vi "Vision Processing.vi"(8 "error in (no error)":errorcluster, 11 "Image Size":T1=enum."320x240") -> ()   [LabVIEW 2017]
uses:
  Vision Support Code/Camera Types.ctl
  <vilib>/Rock Robotics/WPI/Camera/WPI_CameraImageSize.ctl
  <vilib>/Rock Robotics/WPI/Camera/WPI_CameraWhite Balance Values.ctl
  <vilib>/Rock Robotics/WPI/Camera/WPI_CameraExposure Values.ctl
  <vilib>/Rock Robotics/WPI/Camera/WPI_CameraFrameRate.ctl
  Robot Global Data.vi
  <vilib>/Rock Robotics/Network Tables/NT Write Number.vi
  <vilib>/vision/NI_Vision_Development_Module.lvlib
panel:
  in  "max ratio":dbl=8.0 format="%#_13g"
  in  "min ratio":dbl=3.0 format="%#_13g"
  out "error out":errorcluster
  in  "format string":string="USB 0"
  in  "Min Component %":dbl=15.0
  out "loop ms":u32
  in  "Display Original":bool
  in  "Display Mask":bool
  out "Instructions:":string="Connect a USB or IP camera to your roboRIO. If using a ring light and retroreflective tape, use Camera Settings outside the loop create a dark image with bright and colorful stripes. If used wihtout a ring light, brighten the images so that stripes are visible.\n\nLED Color can encoded as HSL or related color modes. Calibrate to the same color as the strips being reflected to the camera. Unlike the desktop example, this LED color must be set by hand. You can also put the calibration on the dashboard and send the LED Color to the RT code using Network Tables.\n\nThe Display buttons affects whether images are displayed on the panel. It takes quite a bit of CPU  to compress and transmit the images for display.\n\nAdjust Score Cutoff to make the code more or less picky. If the color is not very unique, you may need to increase the number of particles considered. The diagram uses a Size Limit to ignore colored things that are too small. You may need to adjust it if you are targetting from far away.\n\nResults give you the distance to the target, the center and box in a normalized (-1 to 1) and pixel coordinates.\n\nBe sure to read about setting camera exposure and brightness to help simplify your image and acquire color saturated images.\n\nThere are lots of comments on the diagram to explain the code."
  in  "Color Mode":u16(ring)=2 items=["RGB", "HSL", "HSV", "HSI"]
  in  "Particles":dbl=5.0
  in  "Score Cutoff %":dbl=75.0
  in  "Camera Type":T2=enum."MS HD3000 square"
  out "Result":T3 {"Score" format="%#_3g"; "Pixels"."Rectangle"."Numeric 5" format="%#_3g"; "Pixels"."Rectangle"."Numeric 3" format="%#_3g"; "Pixels"."Rectangle"."Numeric 2" format="%#_3g"; "Pixels"."Rectangle"."Numeric" format="%#_3g"; "Normalized"."Rectangle"."Numeric 5" format="%#_2g"; "Normalized"."Rectangle"."Numeric 3" format="%#_2g"; "Normalized"."Rectangle"."Numeric 2" format="%#_2g"; "Normalized"."Rectangle"."Numeric" format="%#_2g"; "Normalized"."Center"."?" format="%#_3g"; "Normalized"."Center"."?" format="%#_3g"; "Distance (ft)" format="%#_3g"}
  out "Qualified Particles":i32
  in  "LED Color":T4={"Hue"={107.81818389892578, 139.81818389892578}, "Sat"={176.07142857142858, 255.0}, "Val"={40.53571428571429, 255.0}} {"Hue" scale=0.0..255.0 scale format="%#_3g"}
  out "Mask":T5(plugin-control)
  out "Original Image":T5(plugin-control)
  # "Good target, distance ft"
  # "Bad target"
  # "Score in %"
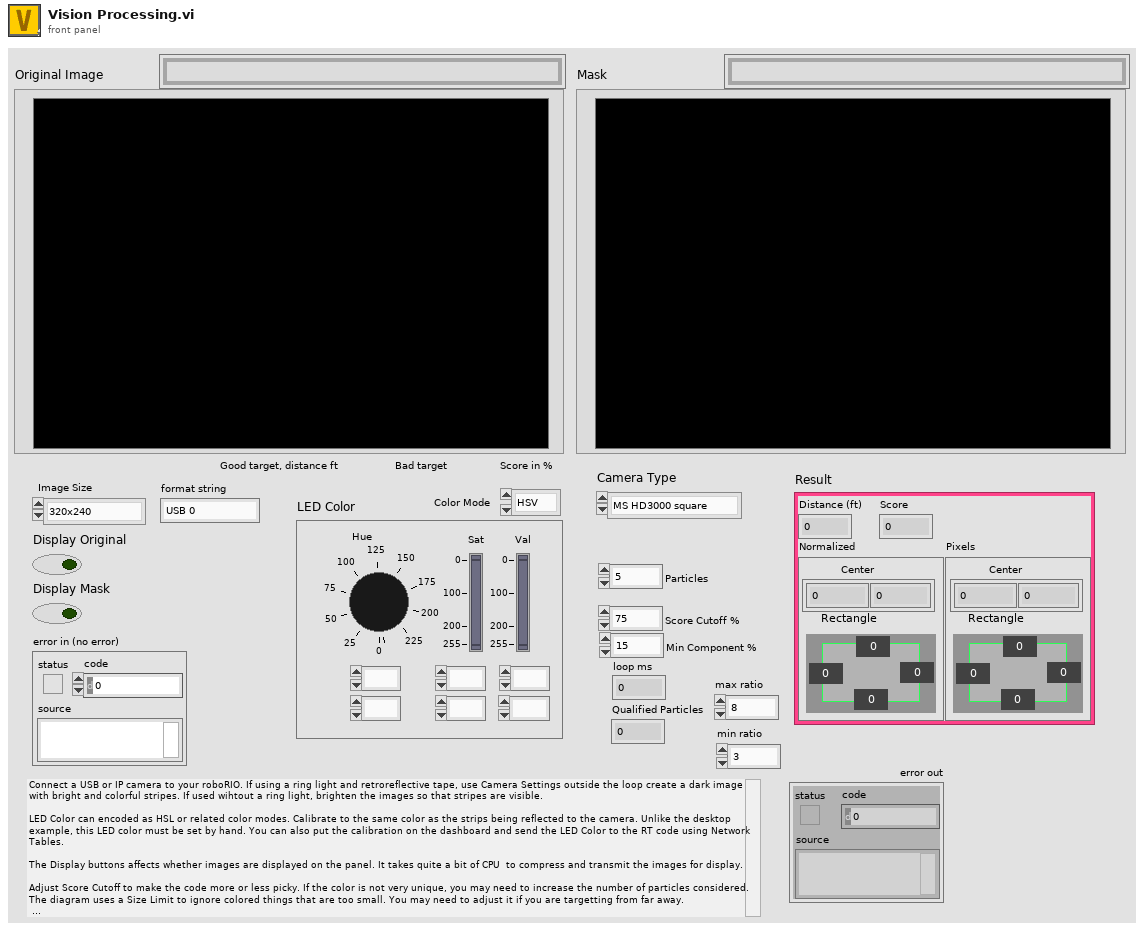
[diagram p1: front panel]
types:
  T1 = typedef "WPI_CameraImageSize.ctl" = enum16{"640x480", "320x240", "160x120", "Custom"}
  T2 = typedef "Camera Types.ctl" = enum16{"206", "1011", "1013", "MS HD3000 square", "MS HD3000 640x480"}
  T3 = cluster{"Distance (ft)":dbl, "Score":dbl, "Normalized":cluster{"Center":cluster{dbl, dbl}, "Rectangle":cluster{"Numeric":dbl, "Numeric 2":dbl, "Numeric 3":dbl, "Numeric 5":dbl}}, "Pixels":cluster{"Center":cluster{dbl, dbl}, "Rectangle":cluster{"Numeric":dbl, "Numeric 2":dbl, "Numeric 3":dbl, "Numeric 5":dbl}}}
  T4 = cluster{"Hue":cluster{dbl, dbl}, "Sat":cluster{dbl, dbl}, "Val":cluster{dbl, dbl}}
  T5 = typedef "IMAQ Image.ctl" = refnum<image>
  T6 = typedef "WPI_CameraFrameRate.ctl" = u32
  T7 = typedef "WPI_CameraExposure Values.ctl" = enum16{"Auto", "Flicker-free 50 Hz", "Flicker-free 60 Hz", "Hold current", "Custom"}
  T8 = typedef "WPI_CameraWhite Balance Values.ctl" = enum16{"Auto", "Fixed indoor", "Fixed outdoor 1", "Fixed outdoor 2", "Fixed fluorescent 1", "Fixed fluorescent 2", "Hold current", "Custom"}
  T9 = typedef "Particle Parameters" = i32
  T10 = typedef "Image Type" = u32
  T11 = typedef "WPI_CameraDevRef.ctl" = cluster{"Camera Address":string, "CameraStatus":errorcluster}
  T12 = cluster{"Score":dbl, "Rect":cluster{"Left":dbl, "Top":dbl, "Right":dbl, "Bottom":dbl}, "Full Scores":cluster{"Aspect Ratio":dbl, "Top Position":dbl, "Bottom Position":dbl, "Left Gap":dbl, "Width":dbl, "Height Ratio":dbl}}[]
  T13 = cluster{"Score":dbl, "Rect":cluster{"Left":dbl, "Top":dbl, "Right":dbl, "Bottom":dbl}, "Full Scores":cluster{"Aspect Ratio":dbl, "Top Position":dbl, "Bottom Position":dbl, "Left Gap":dbl, "Width":dbl, "Height Ratio":dbl}}
  T14 = cluster{"Left":dbl, "Top":dbl, "Right":dbl, "Bottom":dbl}
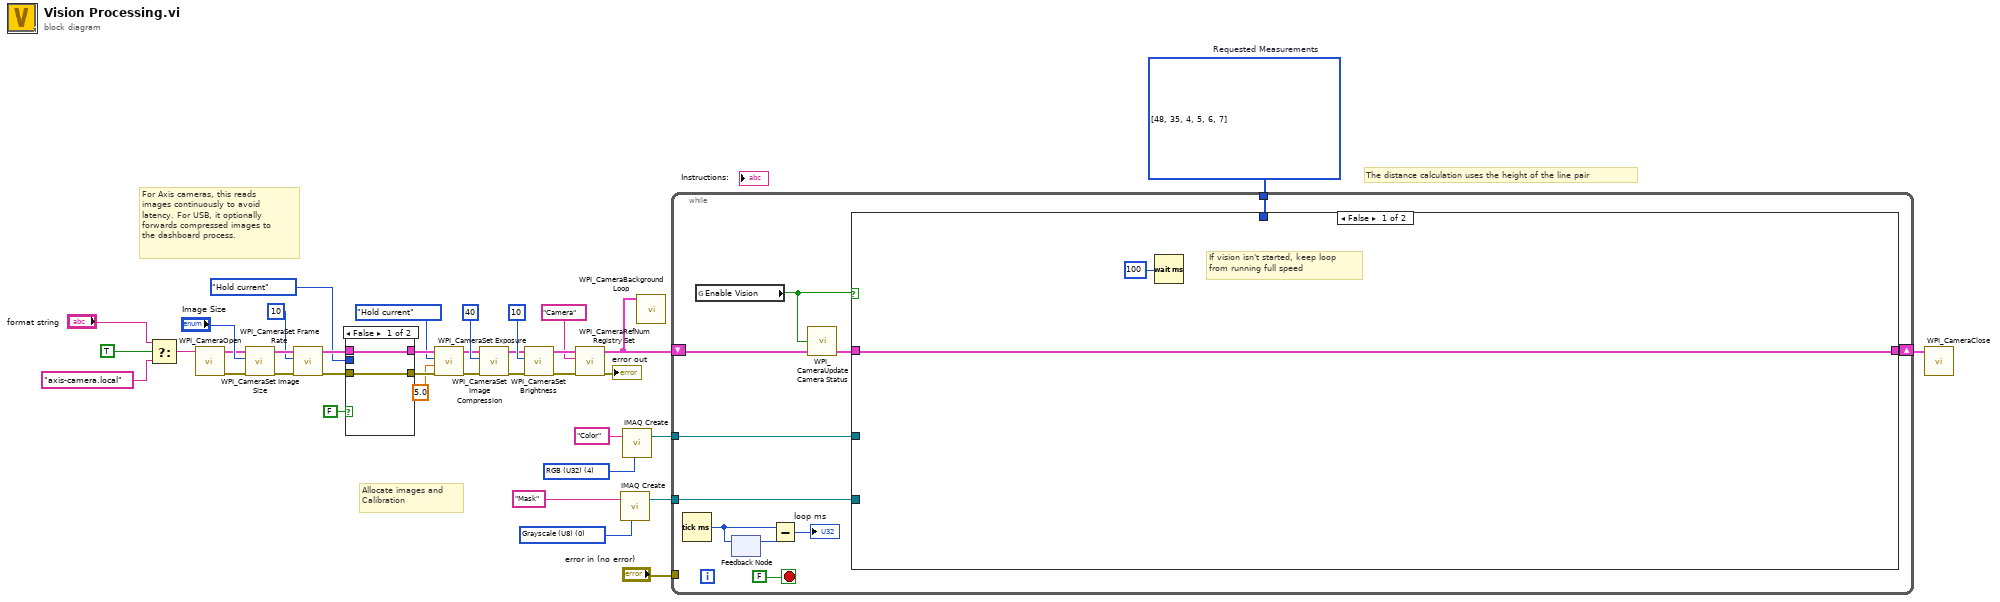
[diagram p0: block diagram]
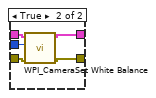
[diagram p2: hidden frame]
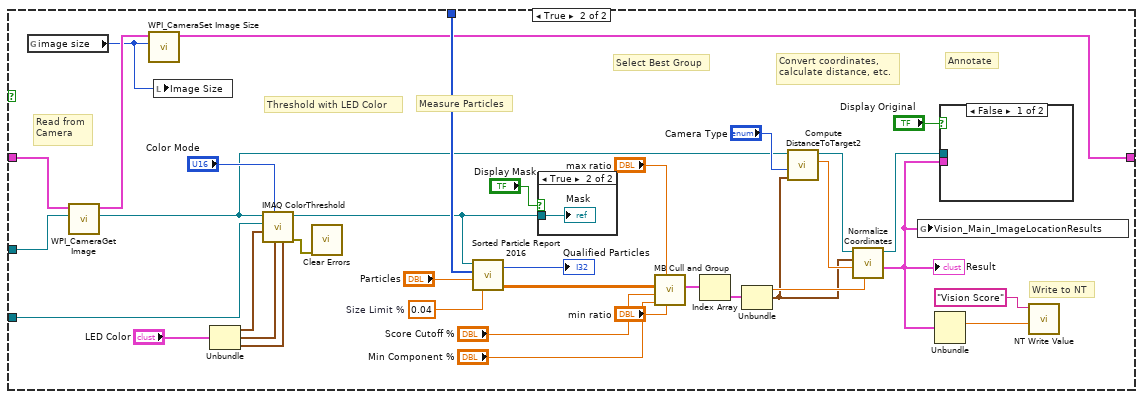
[diagram p3: hidden frame]
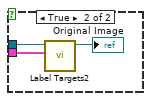
[diagram p4: hidden frame]
diagram:
  w33 = T9[] [48, 35, 4, 5, 6, 7] items=["Center of Mass X", "Center of Mass Y", "First Pixel X", "First Pixel Y", "Bounding Rect Left", "Bounding Rect Top", "Bounding Rect Right", "Bounding Rect Bottom", "Max Feret Diameter Start X", "Max Feret Diameter Start Y", "Max Feret Diameter End X", "Max Feret Diameter End Y", "Max Horiz. Segment Length Left", "Max Horiz. Segment Length Right", "Max Horiz. Segment Length Row", "-", "Bounding Rect Width", "Bounding Rect Height", "Bounding Rect Diagonal", "Perimeter", "Convex Hull Perimeter", "Holes' Perimeter", "Max Feret Diameter", "Equivalent Ellipse Major Axis", "Equivalent Ellipse Minor Axis", "Equivalent Ellipse Minor Axis (Feret)", "Equivalent Rect Long Side", "Equivalent Rect Short Side", "Equivalent Rect Diagonal", "Equivalent Rect Short Side (Feret)", "Average Horiz. Segment Length", "Average Vert. Segment Length", "Hydraulic Radius", "Waddel Disk Diameter", "-", "Area", "Holes' Area", "Particle & Holes' Area", "Convex Hull Area", "Image Area", "-", "Number of Holes", "Number of Horiz. Segments", "Number of Vert. Segments", "-", "Orientation", "Max Feret Diameter Orientation", "-", "% Area/Image Area", "% Area/(Particle & Holes' Area)", "Ratio of Equivalent Ellipse Axes", "Ratio of Equivalent Rect Sides", "-", "Elongation Factor", "Compactness Factor", "Heywood Circularity Factor", "Type Factor", "-", "Sum X", "Sum Y", "Sum XX", "Sum XY", "Sum YY", "Sum XXX", "Sum XXY", "Sum XYY", "Sum YYY", "-", "Moment of Inertia XX", "Moment of Inertia XY", "Moment of Inertia YY", "Moment of Inertia XXX", "Moment of Inertia XXY", "Moment of Inertia XYY", "Moment of Inertia YYY", "Norm. Moment of Inertia XX", "Norm. Moment of Inertia XY", "Norm. Moment of Inertia YY", "Norm. Moment of Inertia XXX", "Norm. Moment of Inertia XXY", "Norm. Moment of Inertia XYY", "Norm. Moment of Inertia YYY", "Hu Moment 1", "Hu Moment 2", "Hu Moment 3", "Hu Moment 4", "Hu Moment 5", "Hu Moment 6", "Hu Moment 7"]  # Requested Measurements
  w36 = T10 0 items=["Grayscale (U8)", "Grayscale (I16)", "Grayscale (SGL)", "Complex (CSG)", "RGB (U32)", "HSL (U32)", "RGB (U64)", "Grayscale (U16)"] ("Image Type")
  w37 = T10 4 items=["Grayscale (U8)", "Grayscale (I16)", "Grayscale (SGL)", "Complex (CSG)", "RGB (U32)", "HSL (U32)", "RGB (U64)", "Grayscale (U16)"] ("Image Type")
  # "For Axis cameras, this reads\nimages continuously to avoid\nlatency. For USB, it optionally\nforwards compressed images to\nthe dashboard process."
  # "The distance calculation uses the height of the line pair"
  # "Allocate images and\nCalibration"
  n1 = Select(t="format string", s=TRUE ("dot notation? (F)"), f="axis-camera.local" ("format string")) -> (s? t:f=w7:string)
  n2 = call <vilib>:"WPI_CameraOpen.vi"("Camera Address"=w7) -> ("error out"=w19:errorcluster, "CameraDevRef"=w20:T11)  [unwired: 1 in, 8 out]
  n3 = call <vilib>:"WPI_CameraSet Image Size.vi"("error in (no error)"=w19, "Image Size"="Image Size", "CameraDevRef"=w20) -> ("error out"=w18:errorcluster, "CameraDevRef Out"=w21:T11)  [unwired: 1 in, 6 out]
  n4 = call <vilib>:"WPI_CameraSet Frame Rate.vi"("error in (no error)"=w18, "Frame Rate (fps)"=T6 10, "CameraDevRef"=w21) -> ("error out"=w17:errorcluster, "CameraDevRef Out"=w23:T11)  [unwired: 7 out]
  n5 = case shown="False" FALSE {
    tunnel: w23 -> [w40 w45]
    tunnel: [w40 w44] -> w22
    tunnel: w17 -> [w39 w43]
    tunnel: [w39 w42] -> w16
    tunnel: WPI_CameraWhite_Balance_Values."Hold current" ("White Balance") -> [_ w41]
    frame False {
    }
    frame True {
      n6 = call <vilib>:"WPI_CameraSet White Balance.vi"("error in (no error)"=w43, "White Balance"=w41, "CameraDevRef"=w45) -> ("error out"=w42:errorcluster, "CameraDevRef Out"=w44:T11)  [unwired: 1 in, 6 out]
    }
  }
  n7 = call <vilib>:"WPI_CameraSet Exposure.vi"("error in (no error)"=w16, "Exposure (%)"=5.0, "Exposure"=WPI_CameraExposure_Values."Hold current", "CameraDevRef"=w22) -> ("error out"=w15:errorcluster, "CameraDevRef Out"=w25:T11)  [unwired: 6 out]
  n8 = call <vilib>:"WPI_CameraSet Image Compression.vi"("error in (no error)"=w15, "Compression"=40, "CameraDevRef"=w25) -> ("error out"=w14:errorcluster, "CameraDevRef Out"=w24:T11)  [unwired: 7 out]
  n9 = call <vilib>:"WPI_CameraSet Brightness.vi"("error in (no error)"=w14, "Brightness"=10, "CameraDevRef"=w24) -> ("error out"=w13:errorcluster, "CameraDevRef Out"=w31:T11)  [unwired: 1 in, 6 out]
  n10 = call <vilib>:"WPI_CameraRefNum Registry Set.vi"("error in (no error)"=w13, "refnum name"="Camera", "CameraDevRef"=w31) -> ("error out"=→"error out":errorcluster, "CameraDevRef"=w6:T11)  [unwired: 1 in, 6 out]
  n11 = call "IMAQ Create"("Image Name"="Mask", "Image Type"=w36) -> ("New Image"=w34:T5)  [unwired: 2 in, 2 out]
  n12 = call "IMAQ Create"("Image Name"="Color", "Image Type"=w37) -> ("New Image"=w32:T5)  [unwired: 2 in, 2 out]
  n13 = call <vilib>:"WPI_CameraBackground Loop.vi"("CameraDevRef"=w6) -> ()  [unwired: 11 in]
  n14 = while {
    tunnel: w32 -> [w53]
    tunnel: w34 -> [w55]
    tunnel: w33 -> [w54]
    shift-right: [w52] -> w5
    shift-left: w6 -> [w51]
    tunnel: "error in (no error)" -> [_]
    stop <- FALSE stop-if-true
    n15 = Tick Count (ms)() -> (millisecond timer value=w47:u32)
    n16 = global read "Robot Global Data.vi" "Enable Vision"() -> (w49:bool)
    n17 = feedback-in #1(w47) -> ()
    n18 = feedback #1() -> (w48:u32)  [unwired: 1 in]
    n19 = Subtract(x=w47, y=w48) -> (x-y=→"loop ms":u32)
    n20 = call <vilib>:"WPI_CameraUpdate Camera Status.vi"("CameraDevRef In"=w51, "Enable Vision"=w49) -> ("CameraDevRef Out"=w50:T11)  [unwired: 3 in]
    n21 = case shown="False" w49 {
      tunnel: w55 -> [_ w94]
      tunnel: w54 -> [_ w90]
      tunnel: w50 -> [w58 w76]
      tunnel: w53 -> [_ w75]
      tunnel: [w58 w70] -> w52
      frame False {
        # "If vision isn't started, keep loop\nfrom running full speed"
        n22 = Wait (ms)(milliseconds to wait=u32 100) -> ()  [unwired: 1 out]
      }
      frame True {
        w88 = 0.04  # Size Limit %
        # "Write to NT"
        # "Read from\nCamera"
        # "Measure Particles"
        # "Convert coordinates,\ncalculate distance, etc."
        # "Annotate"
        # "Select Best Group"
        # "Threshold with LED Color"
        n23 = global read "Robot Global Data.vi" "image size"() -> (w69:T1)
        n24 = call <vilib>:"WPI_CameraGet Image.vi"("Image"=w75, "CameraDevRef"=w76) -> ("Image Out"=w74:T5, "CameraDevRef Out"=w71:T11)  [unwired: 7 in, 1 out]
        n25 = call <vilib>:"WPI_CameraSet Image Size.vi"("Image Size"=w69, "CameraDevRef"=w71) -> ("CameraDevRef Out"=w70:T11)  [unwired: 2 in, 7 out]
        n26 = local write "Image Size"(w69) -> ()
        n27 = Unbundle("LED Color") -> ("Hue"=w93:cluster{dbl, dbl}, "Sat"=w92:cluster{dbl, dbl}, "Val"=w91:cluster{dbl, dbl})
        n28 = call "IMAQ ColorThreshold"("Blue or Luma or Val or Inten Range"=w91, "Green or Sat Range"=w92, "Color Mode"="Color Mode", "Red or Hue Range"=w93, "Image Dst"=w94, "Image Src"=w74) -> ("error out"=w87:errorcluster, "Image Dst Out"=w83:T5)  [unwired: 4 in]
        n29 = call <vilib>:"Clear Errors.vi"("error in (no error)"=w87) -> ()  [unwired: 5 in, 2 out]
        n30 = call "Sorted Particle Report 2016.vi"("Min Area Size %"=w88, "Particle Count Limit"="Particles", "Pixel Measurements"=w90, "Image in"=w83) -> ("Sorted Data"=w85:dbl[][], "Particles"=→"Qualified Particles":i32)
        n31 = case shown="True" "Display Mask" {
          tunnel: w83 -> [_ w98]
          frame False {
          }
          frame True {
            "Mask" <- w98
          }
        }
        n32 = call "MB Cull and Group.vi"("min ratio"="min ratio", "max ratio"="max ratio", "Max"="Min Component %", "min"="Score Cutoff %", "Sorted Data"=w85) -> ("Best Targets above cutoff"=w65:T12)  [unwired: 6 in]
        n33 = Index Array(array=w65) -> (element=w64:T13)  [unwired: 1 in]
        n34 = Unbundle(w64) -> ("Score"=w63:dbl, "Rect"=w62:T14)  [unwired: 1 out]
        n35 = call "Compute DistanceToTarget2.vi"("Rect"=w62, "Camera Type"="Camera Type", "Image Src"=w74) -> ("Distance (ft)"=w81:dbl, "Image Dst Out"=w80:T5)  [unwired: 7 in]
        n36 = call "Normalize Coordinates.vi"("Score"=w63, "Distance"=w81, "Bounding box"=w62, "Image in"=w80) -> ("Results"=w68:T3, "Image out"=w79:T5)  [unwired: 6 in]
        "Result" <- w68
        n37 = global write "Robot Global Data.vi" "Vision_Main_ImageLocationResults"(w68) -> ()
        n38 = Unbundle(w68) -> ("Score"=w67:dbl)  [unwired: 3 out]
        n39 = case shown="False" "Display Original" {
          tunnel: w79 -> [_ w96]
          tunnel: w68 -> [_ w95]
          frame False {
          }
          frame True {
            n40 = call "Label Targets2.vi"("Results"=w95, "Image in"=w96) -> ("Image out"=→"Original Image":T5)  [unwired: 9 in]
          }
        }
        n41 = call-poly <vilib>:"NT Write Value.vi"("Numeric"=w67, "Name"="Vision Score") -> ()  [unwired: 9 in, 1 out]
      }
    }
  }
  n42 = call <vilib>:"WPI_CameraClose.vi"("CameraDevRef"=w5) -> ()  [unwired: 1 in, 10 out]
